vi "Page Project.vi"() -> ()   [LabVIEW 2018, in "Main.lvlib"]
uses:
  Main.lvlib
panel:
  in  "Project Lbx":i32(listbox)=-1 caption="Project"
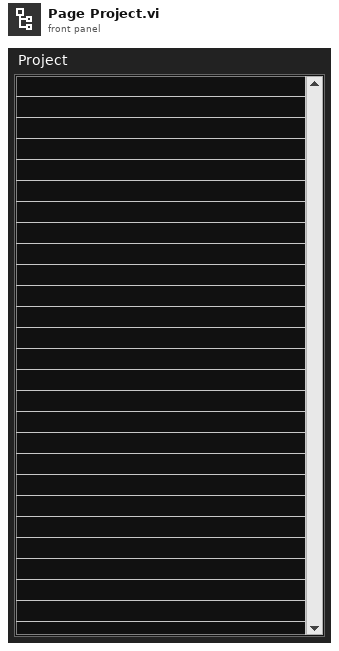
[diagram p1: front panel]
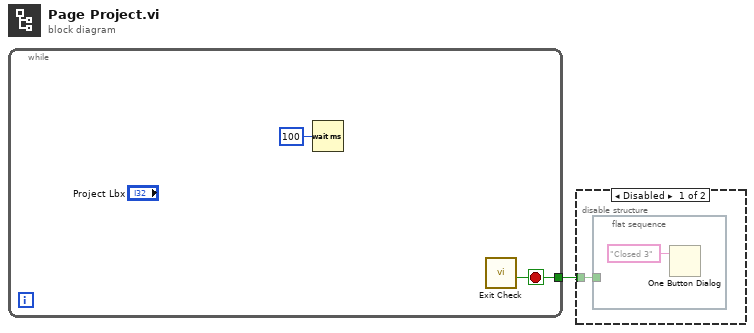
[diagram p0: block diagram]
diagram:
  n1 = while {
    tunnel: [w2] -> w1
    stop <- w2 stop-if-true
    n2 = Wait (ms)(milliseconds to wait=u32 100) -> ()  [unwired: 1 out]
    n3 = call "Exit Check.vi"() -> ("Exit?"=w2:bool)  [unwired: 10 in, 1 out]
  }
  n4 = disable-structure shown="Disabled" {
    disable-tunnel: w1 -> [w4 _]
    frame Disabled {
      n5 = flat-sequence {
        tunnel: w4 -> [_]
        frame #0 {
          n6 = One Button Dialog(message="Closed 3") -> ()  [unwired: 1 in, 1 out]
        }
      }
    }
    frame Enabled {
    }
  }
